vi "decode multi-part content.vi"(8 "error in (no error)":errorcluster, 10 "Valid Content-Type: (\"text/xml\")":string="text/xml", 11 "Multi-Part Content (\"\")":string) -> (0 "error out":errorcluster, 3 "Content":string)   [LabVIEW 2011]
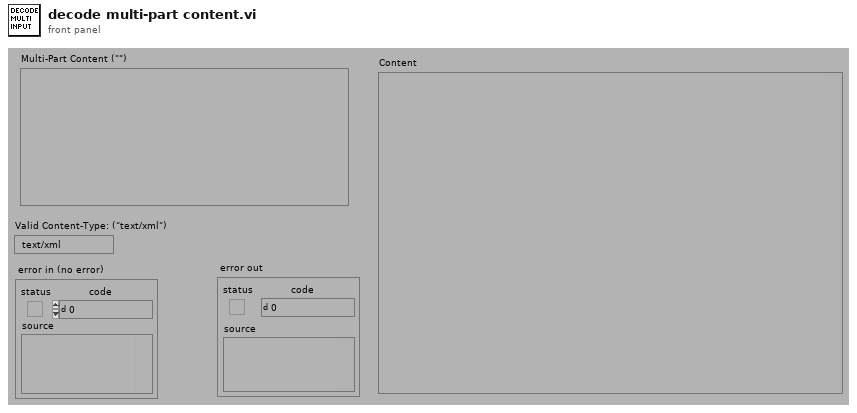
[diagram p1: front panel]
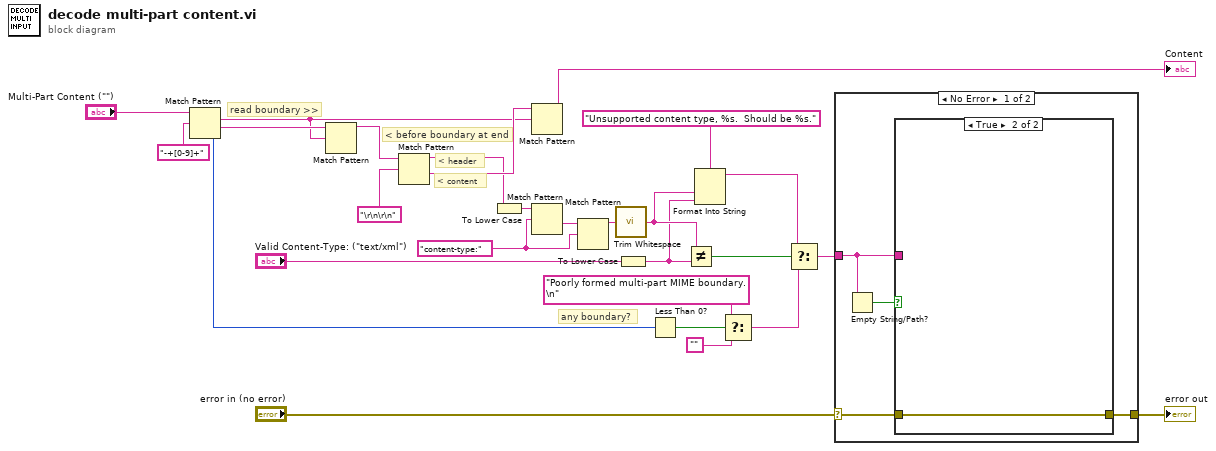
[diagram p0: block diagram]
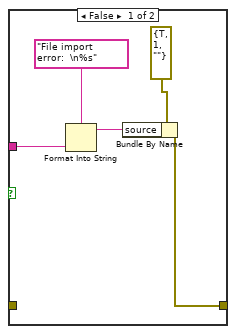
[diagram p2: hidden frame]
diagram:
  w16 = "content-type:" ("regular expression")
  # "any boundary?"
  # "< header"
  # "< content"
  # "< before boundary at end"
  # "read boundary >>"
  n1 = Match Pattern(string="Multi-Part Content (\"\")", regular expression="-+[0-9]+") -> (match substring=w19:string, after substring=w20:string, offset past match=w23:i32)  [unwired: 2 out]
  n2 = Match Pattern(string=w20, regular expression=w19) -> (before substring=w1:string)  [unwired: 4 out]
  n3 = Match Pattern(string=w1, regular expression="\r\n\r\n") -> (before substring=w18:string, after substring=w25:string)  [unwired: 3 out]
  n4 = To Lower Case(string=w18) -> (all lower case string=w21:string)
  n5 = Match Pattern(string=w25, regular expression=w19) -> (before substring=→"Content":string)  [unwired: 4 out]
  n6 = Match Pattern(string=w21, regular expression=w16) -> (after substring=w17:string)  [unwired: 4 out]
  n7 = Match Pattern(string=w17, regular expression=w16) -> (before substring=w15:string)  [unwired: 4 out]
  n8 = call <vilib>:"Trim Whitespace.vi"("string"=w15) -> ("trimmed string"=w11:string)  [unwired: 1 in]
  n9 = To Lower Case(string="Valid Content-Type: (\"text/xml\")") -> (all lower case string=w10:string)
  n10 = Less Than 0?(x=w23) -> (x < 0?=w8:bool)
  n11 = Not Equal?(x=w11, y=w10) -> (x != y?=w13:bool)
  n12 = Format Into String(format string="Unsupported content type, %s.  Should be %s." ("source"), w11, w10) -> (resulting string=w9:string)  [unwired: 2 in, 1 out]
  n13 = Select(t="Poorly formed multi-part MIME boundary.\n" ("source"), s=w8, f="") -> (s? t:f=w6:string)
  n14 = Select(t=w9, s=w13, f=w6) -> (s? t:f=w4:string)
  n15 = case shown="No Error" "error in (no error)" {
    selector: "error in (no error)" -> [w31 w38]
    tunnel: [w28 w38] -> w14
    tunnel: w4 -> [w29 _]
    frame No Error {
      n16 = Empty String/Path?(string/path=w29) -> (empty?=w30:bool)
      n17 = case shown="True" w30 {
        tunnel: w31 -> [_ w37]
        tunnel: w29 -> [w33 _]
        tunnel: [w32 w37] -> w28
        frame False {
          n18 = Format Into String(format string="File import error:  \n%s" ("source"), w33) -> (resulting string=w34:string)  [unwired: 2 in, 1 out]
          n19 = Bundle By Name(cluster=errorcluster {"status"=TRUE, "code"=1, "source"=""} ("t"), "source"=w34) -> (w32:errorcluster)
        }
        frame True {
        }
      }
    }
    frame Error {
    }
  }
  "error out" <- w14
